vi "Read Injector Event Count from FPGA.vi"(8 "error in (no error)":errorcluster, 10 "Injector index":i16, 11 "FPGA Reference":T1) -> (0 "error out":errorcluster, 2 "Injector Event Count":u32)   [LabVIEW 2015, in "Fuel Injection Addon Engine.lvlib"]
uses:
  Fuel Injection Addon Engine.lvlib
  Types/FPGA Reference.ctl
  <vilib>/Utility/error.llb/Error Cluster From Error Code.vi
  <vilib>/rvi/errors/niLvFpgaAdjustHostInterfaceError.vi
  <vilib>/rvi/interface/nirviReadWriteControl/nirviReadWriteControl.xnode
  NiFpgaLv.dll
  <vilib>/rvi/interface/Simulation/niFpgaSimulationCallBeginRW.vi
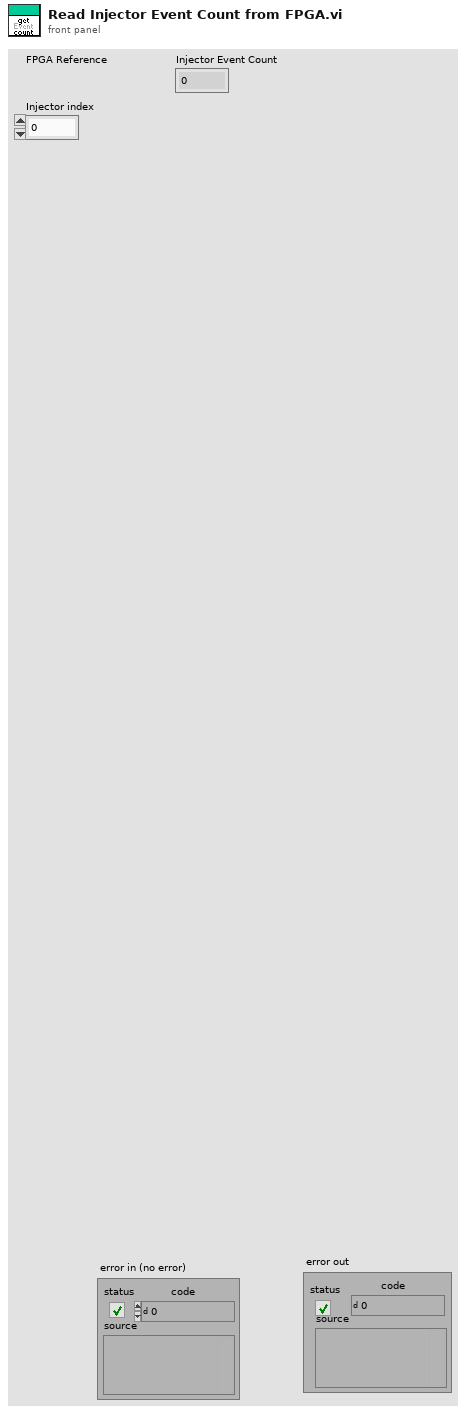
[diagram p1: front panel]
types:
  T1 = typedef "Fuel Injection Addon Engine.lvlib/FPGA Reference.ctl" = refnum<k20>
  T2 = cluster{"Injector 1":u32, "Injector 2":u32, "Injector 3":u32, "Injector 4":u32, "Injector 5":u32, "Injector 6":u32, "Injector 7":u32, "Injector 8":u32, "Injector 9":u32, "Injector 10":u32, "Injector 11":u32, "Injector 12":u32, "Injector 13":u32, "Injector 14":u32, "Injector 15":u32, "Injector 16":u32}
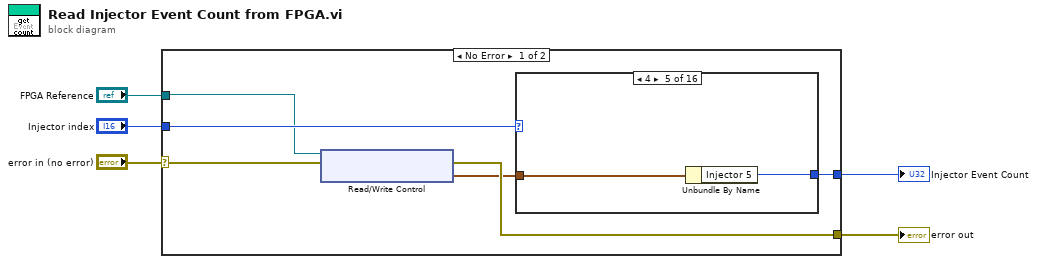
[diagram p0: block diagram]
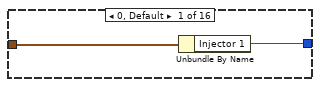
[diagram p2: hidden frame]
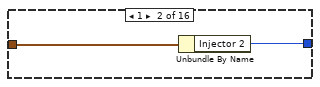
[diagram p3: hidden frame]
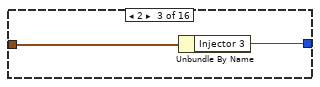
[diagram p4: hidden frame]
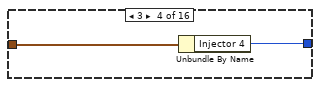
[diagram p5: hidden frame]
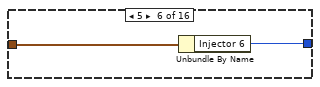
[diagram p6: hidden frame]
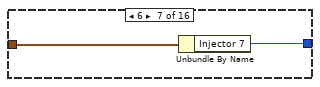
[diagram p7: hidden frame]
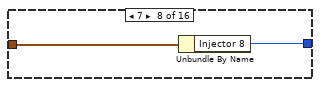
[diagram p8: hidden frame]
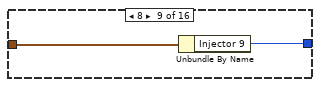
[diagram p9: hidden frame]
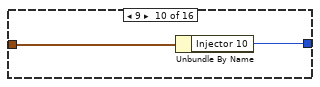
[diagram p10: hidden frame]
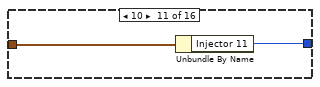
[diagram p11: hidden frame]
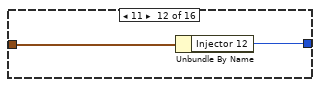
[diagram p12: hidden frame]
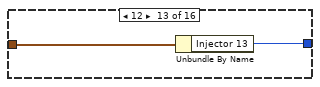
[diagram p13: hidden frame]
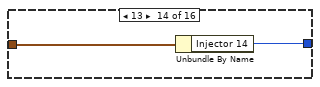
[diagram p14: hidden frame]
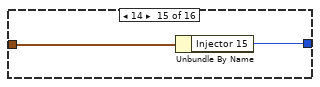
[diagram p15: hidden frame]
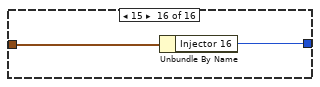
[diagram p16: hidden frame]
diagram:
  n1 = case shown="No Error" "error in (no error)" {
    selector: "error in (no error)" -> [w8 w44]
    tunnel: "Injector index" -> [w11 _]
    tunnel: [w7 w44] -> w4
    tunnel: [w10 _] -> w2
    tunnel: "FPGA Reference" -> [w9 _]
    frame No Error {
      n2 = xnode "Read/Write Control"("FPGA VI Reference In"=w9, "error in"=w8) -> ("error out"=w7:errorcluster, "Event Capture Cluster"=w6:T2)  [unwired: 1 out]
      n3 = case shown="4" w11 {
        tunnel: w6 -> [w13 w15 w17 w19 w21 w23 w25 w27 w29 w31 w33 w35 w37 w39 w41 w42]
        tunnel: [w12 w14 w16 w18 w20 w22 w24 w26 w28 w30 w32 w34 w36 w38 w40 w43] -> w10
        frame 0, Default {
          n4 = Unbundle By Name(w13) -> ("Injector 1"=w12:u32)
        }
        frame 1 {
          n5 = Unbundle By Name(w15) -> ("Injector 2"=w14:u32)
        }
        frame 2 {
          n6 = Unbundle By Name(w17) -> ("Injector 3"=w16:u32)
        }
        frame 3 {
          n7 = Unbundle By Name(w19) -> ("Injector 4"=w18:u32)
        }
        frame 4 {
          n8 = Unbundle By Name(w21) -> ("Injector 5"=w20:u32)
        }
        frame 5 {
          n9 = Unbundle By Name(w23) -> ("Injector 6"=w22:u32)
        }
        frame 6 {
          n10 = Unbundle By Name(w25) -> ("Injector 7"=w24:u32)
        }
        frame 7 {
          n11 = Unbundle By Name(w27) -> ("Injector 8"=w26:u32)
        }
        frame 8 {
          n12 = Unbundle By Name(w29) -> ("Injector 9"=w28:u32)
        }
        frame 9 {
          n13 = Unbundle By Name(w31) -> ("Injector 10"=w30:u32)
        }
        frame 10 {
          n14 = Unbundle By Name(w33) -> ("Injector 11"=w32:u32)
        }
        frame 11 {
          n15 = Unbundle By Name(w35) -> ("Injector 12"=w34:u32)
        }
        frame 12 {
          n16 = Unbundle By Name(w37) -> ("Injector 13"=w36:u32)
        }
        frame 13 {
          n17 = Unbundle By Name(w39) -> ("Injector 14"=w38:u32)
        }
        frame 14 {
          n18 = Unbundle By Name(w41) -> ("Injector 15"=w40:u32)
        }
        frame 15 {
          n19 = Unbundle By Name(w42) -> ("Injector 16"=w43:u32)
        }
      }
    }
    frame Error {
    }
  }
  "error out" <- w4
  "Injector Event Count" <- w2
